vi "Battery Dispatch.vi"() -> ()   [LabVIEW 2016]
panel:
  in  "BatteryDispatch":dbl[](array[numeric])
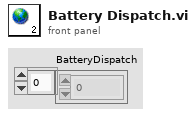
[diagram p1: front panel]
diagram:
